vi "updateEnt_logHistSeq.vi"() -> ()   [LabVIEW 2012]
uses:
  <vilib>/addons/database/Connection.llb/DB Tools Open Connec (Path).vi
  <vilib>/addons/database/Connection.llb/Conn Execute.vi
  <vilib>/addons/database/Recordset.llb/Rec Destroy - Connection.vi
  <vilib>/addons/database/Recordset.llb/Rec Fetch Recordset Data (R).vi
  <vilib>/addons/database/_DB Variant To Data/Database Variant To Data.xnode
  <vilib>/addons/database/NI_Database_API.lvlib
panel:
  out "error out 2":errorcluster
  out "concatenated string 2":string
  out "error out 4":errorcluster
  out "error out 3":errorcluster
  out "SQL query":string="select  distinct ent_entity,MAX(ent_hist_seq), from ems.dbo.ent_log_TMP \ngroup by ent_entity\norder by ent_entity "
  out "recordset data":variant[][](array[variant])
  out "error out":errorcluster
  out "result":i32
  out "concatenated string":string
  out "recordset data 2":variant[][](array[variant])
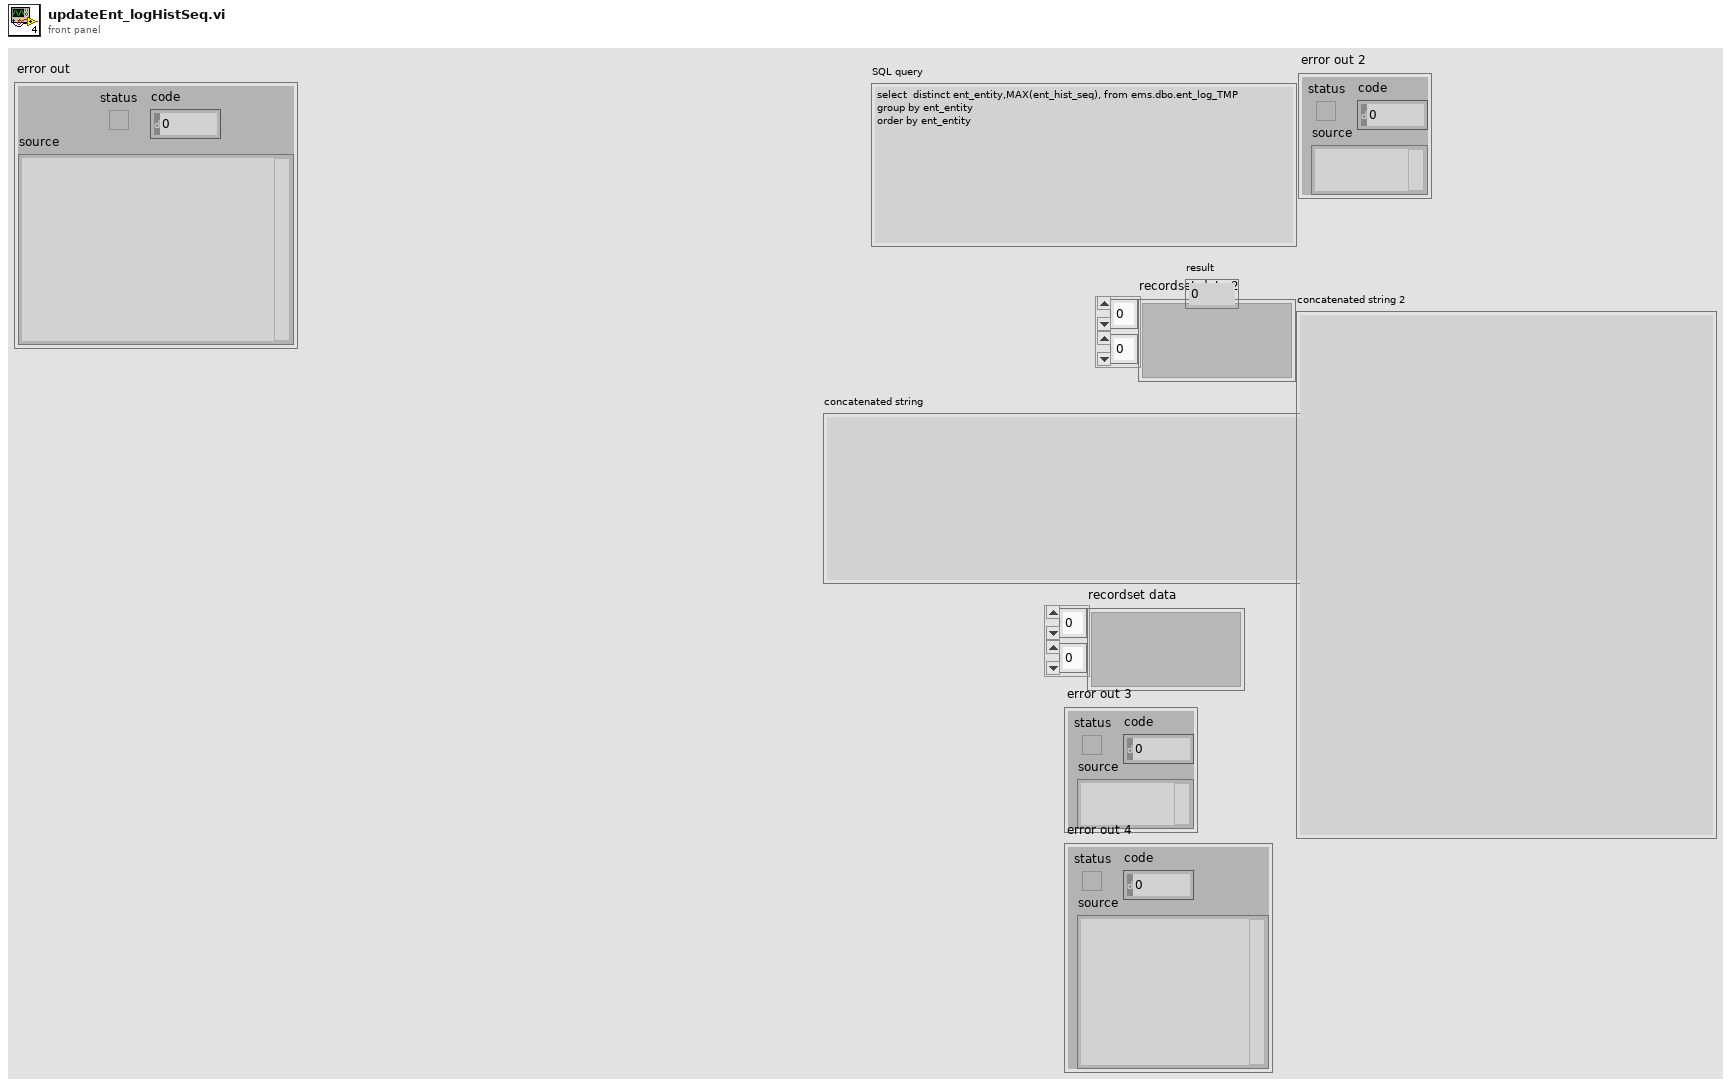
[diagram p1: front panel]
types:
  T1 = typedef "NI_Database_API.lvlib/Conn ObjectReference.ctl" = refnum<k1>
  T2 = typedef "NI_Database_API.lvlib/Rec ObjectReference.ctl" = refnum<k1>
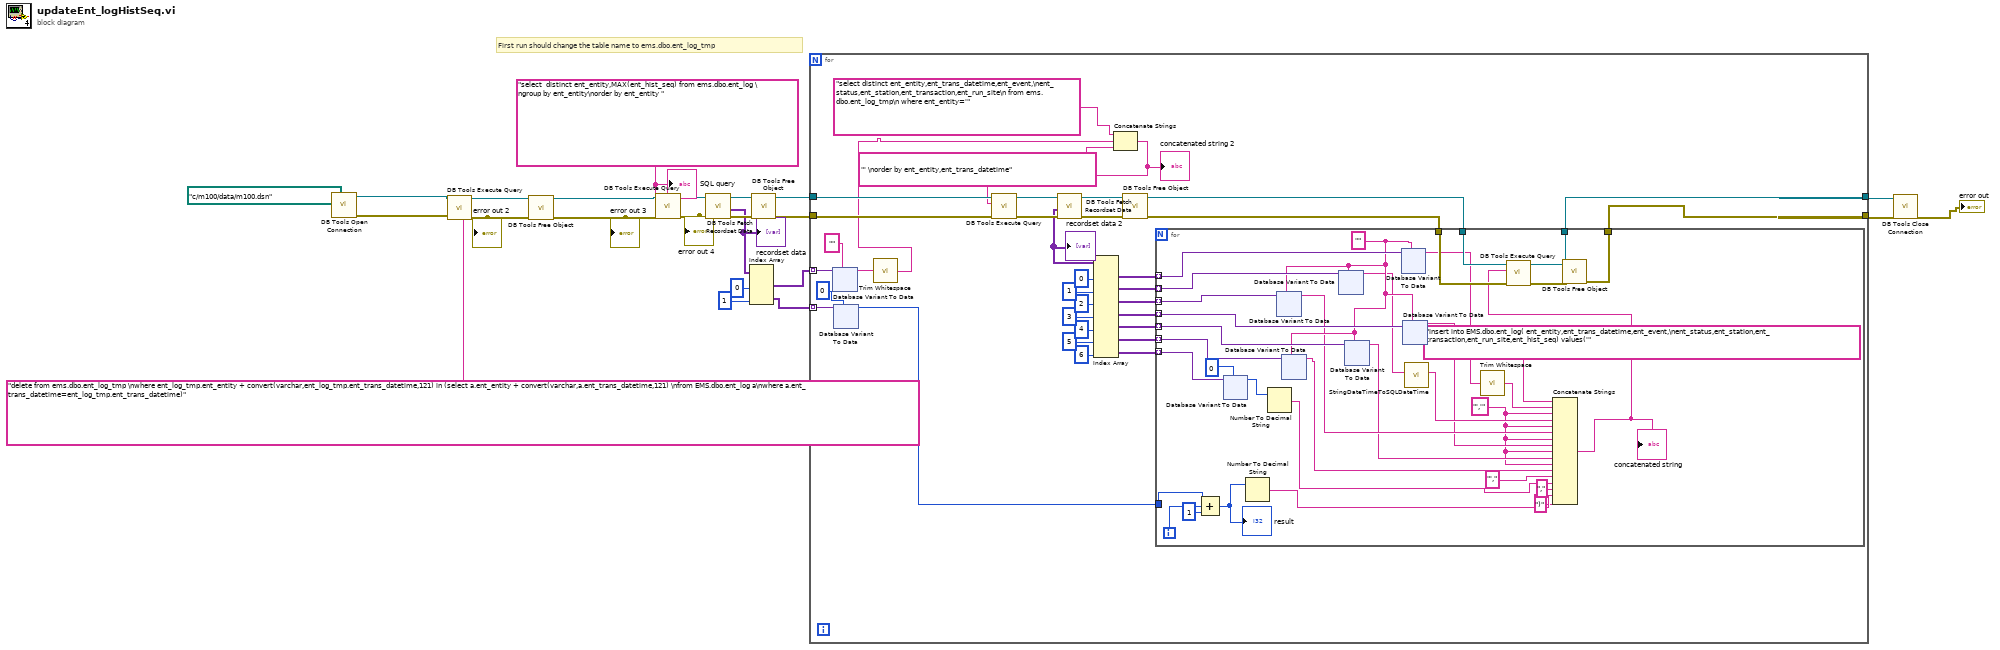
[diagram p0: block diagram]
diagram:
  w16 = "select  distinct ent_entity,MAX(ent_hist_seq) from ems.dbo.ent_log \ngroup by ent_entity\norder by ent_entity " ("SQL query")
  # "First run should change the table name to ems.dbo.ent_log_tmp"
  n1 = call-poly <vilib>:"DB Tools Open Connection.vi"("connection information"=path "c:/m100/data/m100.dsn") -> ("error out"=w7:errorcluster, "connection reference"=w10:T1)  [unwired: 7 in]
  n2 = call-poly <vilib>:"DB Tools Execute Query.vi"("error in (no error)"=w7, "SQL query"="delete from ems.dbo.ent_log_tmp \nwhere ent_log_tmp.ent_entity + convert(varchar,ent_log_tmp.ent_trans_datetime,121) in (select a.ent_entity + convert(varchar,a.ent_trans_datetime,121) \nfrom EMS.dbo.ent_log a\nwhere a.ent_trans_datetime=ent_log_tmp.ent_trans_datetime)", "connection reference"=w10) -> ("error out"=w6:errorcluster, "recordset reference"=w9:T2)  [unwired: 5 in]
  "error out 2" <- w6
  n3 = call-poly <vilib>:"DB Tools Free Object.vi"("error in (no error)"=w6, "recordset reference"=w9) -> ("error out"=w5:errorcluster, "connection reference"=w8:T1)  [unwired: 8 in]
  "error out 3" <- w5
  n4 = call-poly <vilib>:"DB Tools Execute Query.vi"("error in (no error)"=w5, "SQL query"=w16, "connection reference"=w8) -> ("error out"=w17:errorcluster, "recordset reference"=w22:T2)  [unwired: 5 in]
  "error out 4" <- w17
  n5 = call-poly <vilib>:"DB Tools Fetch Recordset Data.vi"("error in (no error)"=w17, "recordset reference"=w22) -> ("error out"=w18:errorcluster, "recordset data"=w15:variant[][], "recordset reference out"=w21:T2)  [unwired: 3 in]
  "recordset data" <- w15
  n6 = Index Array(array=w15, index (col) #1=0 ("disabled index (col)"), index (col) #2=1 ("index (col)")) -> (element #1=w13:variant[], element #2=w11:variant[])  [unwired: 2 in]
  n7 = call-poly <vilib>:"DB Tools Free Object.vi"("error in (no error)"=w18, "recordset reference"=w21) -> ("error out"=w19:errorcluster, "connection reference"=w20:T1)  [unwired: 8 in]
  n8 = for {
    tunnel: w20 -> [w41]
    tunnel: w19 -> [w40]
    tunnel: w13 -> [w38] mode=indexing
    tunnel: [w27] -> w2
    tunnel: [w26] -> w1
    tunnel: w11 -> [w32] mode=indexing
    n9 = xnode "Database Variant To Data"("database variant"=w38, "type"="") -> ("data"=w35:string)  [unwired: 1 in, 1 out]
    n10 = xnode "Database Variant To Data"("database variant"=w32, "type"=0) -> ("data"=w24:i32)  [unwired: 1 in, 1 out]
    n11 = call <vilib>:"Trim Whitespace.vi"("string"=w35) -> ("trimmed string"=w33:string)  [unwired: 1 in]
    n12 = Concatenate Strings("select distinct ent_entity,ent_trans_datetime,ent_event,\nent_status,ent_station,ent_transaction,ent_run_site\n from ems.dbo.ent_log_tmp\n where ent_entity='" ("SQL query"), w33, "' \norder by ent_entity,ent_trans_datetime" ("string")) -> (w36:string)
    "concatenated string 2" <- w36
    n13 = call-poly <vilib>:"DB Tools Execute Query.vi"("error in (no error)"=w40, "SQL query"=w36, "connection reference"=w41) -> ("error out"=w56:errorcluster, "recordset reference"=w58:T2)  [unwired: 5 in]
    n14 = call-poly <vilib>:"DB Tools Fetch Recordset Data.vi"("error in (no error)"=w56, "recordset reference"=w58) -> ("error out"=w55:errorcluster, "recordset data"=w30:variant[][], "recordset reference out"=w57:T2)  [unwired: 3 in]
    "recordset data 2" <- w30
    n15 = Index Array(array=w30, index (col) #1=0 ("disabled index (col)"), index (col) #2=1 ("index (col)"), index (col) #3=2 ("index (col)"), index (col) #4=3 ("index (col)"), index (col) #5=4 ("index (col)"), index (col) #6=5 ("index (col)"), index (col) #7=6 ("index (col)")) -> (element #1=w47:variant[], element #2=w46:variant[], element #3=w45:variant[], element #4=w39:variant[], element #5=w44:variant[], element #6=w43:variant[], element #7=w42:variant[])  [unwired: 7 in]
    n16 = call-poly <vilib>:"DB Tools Free Object.vi"("error in (no error)"=w55, "recordset reference"=w57) -> ("error out"=w28:errorcluster, "connection reference"=w29:T1)  [unwired: 8 in]
    n17 = for {
      tunnel: w47 -> [w158] mode=indexing
      tunnel: w46 -> [w157] mode=indexing
      tunnel: w45 -> [w156] mode=indexing
      tunnel: w44 -> [w154] mode=indexing
      tunnel: w39 -> [w155] mode=indexing
      tunnel: w43 -> [w153] mode=indexing
      tunnel: w42 -> [w152] mode=indexing
      tunnel: w29 -> [w149]
      tunnel: w28 -> [w148]
      tunnel: [w151] -> w27
      tunnel: [w150] -> w26
      tunnel: w24 -> [w137]
      i -> [w145]
      w131 = "','" ("string")
      w143 = ""
      n18 = Compound Arithmetic op=ADD(w137, w145, 1 ("value")) -> (w140:i32)
      "result" <- w140
      n19 = xnode "Database Variant To Data"("database variant"=w152, "type"=0) -> ("data"=w127:i32)  [unwired: 1 in, 1 out]
      n20 = Number To Decimal String(number=w140) -> (decimal integer string=w124:string)  [unwired: 1 in]
      n21 = Number To Decimal String(number=w127) -> (decimal integer string=w126:string)  [unwired: 1 in]
      n22 = xnode "Database Variant To Data"("database variant"=w156, "type"=w143) -> ("data"=w134:string)  [unwired: 1 in, 1 out]
      n23 = xnode "Database Variant To Data"("database variant"=w153, "type"=w143) -> ("data"=w130:string)  [unwired: 1 in, 1 out]
      n24 = xnode "Database Variant To Data"("database variant"=w157, "type"=w143) -> ("data"=w139:string)  [unwired: 1 in, 1 out]
      n25 = xnode "Database Variant To Data"("database variant"=w154, "type"=w143) -> ("data"=w132:string)  [unwired: 1 in, 1 out]
      n26 = xnode "Database Variant To Data"("database variant"=w158, "type"=w143) -> ("data"=w138:string)  [unwired: 1 in, 1 out]
      n27 = xnode "Database Variant To Data"("database variant"=w155, "type"=w143) -> ("data"=w133:string)  [unwired: 1 in, 1 out]
      n28 = call "StringDateTimeToSQLDateTime.vi"("String"=w139) -> ("date/time string"=w135:string)  [unwired: 9 in, 1 out]
      n29 = call <vilib>:"Trim Whitespace.vi"("string"=w138) -> ("trimmed string"=w136:string)  [unwired: 1 in]
      n30 = Concatenate Strings("insert into EMS.dbo.ent_log( ent_entity,ent_trans_datetime,ent_event,\nent_status,ent_station,ent_transaction,ent_run_site,ent_hist_seq) values('", w136, w131, w135, w131, w134, w131, w133, w131, w132, w131, w130, "'," ("string"), w126, "," ("string"), w124, ")" ("string")) -> (w142:string)
      "concatenated string" <- w142
      n31 = call-poly <vilib>:"DB Tools Execute Query.vi"("error in (no error)"=w148, "SQL query"=w142, "connection reference"=w149) -> ("error out"=w146:errorcluster, "recordset reference"=w147:T2)  [unwired: 5 in]
      n32 = call-poly <vilib>:"DB Tools Free Object.vi"("error in (no error)"=w146, "recordset reference"=w147) -> ("error out"=w150:errorcluster, "connection reference"=w151:T1)  [unwired: 8 in]
    }
  }
  n33 = call <vilib>:"DB Tools Close Connection.vi"("error in (no error)"=w1, "connection reference"=w2) -> ("error out"=→"error out":errorcluster)  [unwired: 5 in]
  "SQL query" <- w16
